vi "Get All Property Names.vi"(8 "error in":errorcluster, 11 "Item in":refnum<class "Item.lvclass">) -> (0 "error out":errorcluster, 3 "Property Names":string[](array[string]))   [LabVIEW 2024, in "Parser.lvlib" / "Property.lvclass"]
uses:
  Property.lvclass
  Property.lvclass/Property.ctl
  Item/Item.lvclass
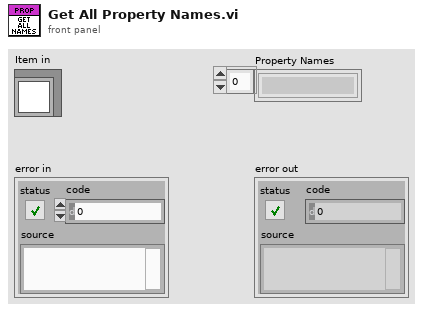
[diagram p1: front panel]
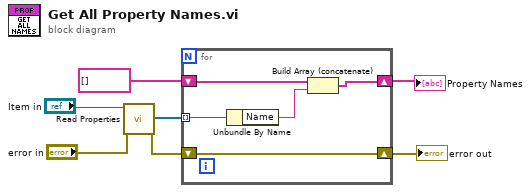
[diagram p0: block diagram]
diagram:
  n1 = call "Read Properties.vi"("error in"="error in", "Item in"="Item in") -> ("error out"=w6:errorcluster, "Properties"=w2:refnum<class "Property.lvclass">[])  [unwired: 7 in, 1 out]
  n2 = for {
    tunnel: w2 -> [w11] mode=indexing
    shift-right: [w12] -> w7
    shift-left: w6 -> [w12]
    shift-right: [w9] -> w3
    shift-left: string[] [] -> [w10]
    n3 = Unbundle By Name(w11) -> ("Name"=w8:string)
    n4 = Build Array (concatenate)(w10, w8) -> (w9:string[])
  }
  "error out" <- w7
  "Property Names" <- w3
